vi "ATMonochromator_issueCommand_selectGrating.vi"(8 "error in (no error)":errorcluster, 11 "command_selectGrating_Ctl":T1) -> (0 "error out":errorcluster, 2 "function return":i32, 3 "command_selectGrating_Ctl out":T1)   [LabVIEW 2016, in "SALLV_ATMonochromator.lvlib"]
doc: "int ATMonochromator_shm_issueCommand_selectGratingLV(ATMonochromator_command_selectGratingLV *command_selectGrating_Ctl );"
uses:
  SALLV_ATMonochromator.lvlib
  DataTypes/command_selectGrating.ctl
  SALLV_ATMonochromator.so
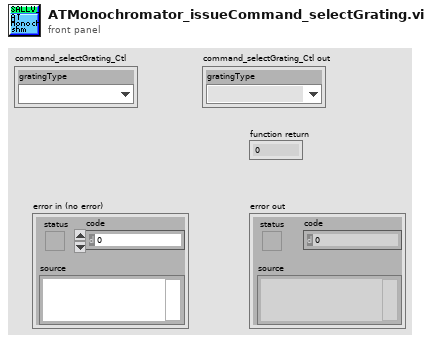
[diagram p1: front panel]
types:
  T1 = typedef "SALLV_ATMonochromator.lvlib/command_selectGrating.ctl" = cluster{"gratingType":enum32{"", "Blue", "Red", "Mirror"}}
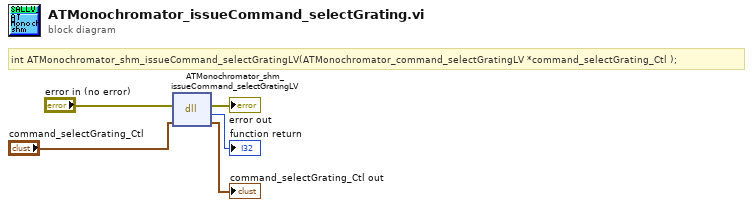
[diagram p0: block diagram]
diagram:
  # "int ATMonochromator_shm_issueCommand_selectGratingLV(ATMonochromator_command_selectGratingLV *command_selectGrating_Ctl );"
  n1 = dll-call lib="home/harini/tcs/SALLV_ATMonochromator/SALLV_ATMonochromator.*" fn="ATMonochromator_shm_issueCommand_selectGratingLV"(error in="error in (no error)", "command_selectGrating_Ctl"="command_selectGrating_Ctl") -> (error out=→"error out":errorcluster, →"function return":i32, "command_selectGrating_Ctl"=→"command_selectGrating_Ctl out":T1)  [unwired: 2 in, 1 out]
